vi "Execution_LaunchAnyProcess.vi"(7 "EVE reference in":refnum<data-value>, 8 "error in (no error)":errorcluster, 11 "Process in":refnum<class "Process.lvclass">) -> (0 "error out":errorcluster, 2 "vi reference":refnum<vi>, 3 "Process out":refnum<class "Process.lvclass">)   [LabVIEW 2013, in "Process.lvclass"]
uses:
  Process.lvclass
  001 - MAIN/Class/EVE/EVE.lvclass
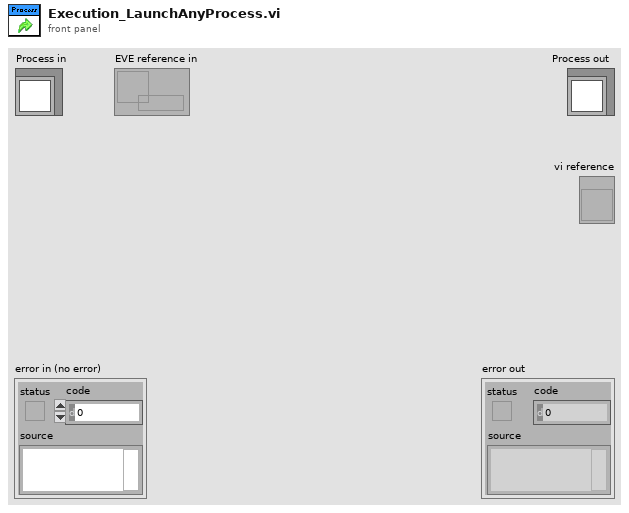
[diagram p1: front panel]
types:
  T1 = typedef "paramsExternalProcesses.ctl" = cluster{"Path":path, "Timeout":dbl, "viInitString":string, "State":enum32{"Invalid", "Standard", "Closed", "Hidden", "Minimized", "Maximized"}}
  T2 = enum32{"Invalid", "Standard", "Closed", "Hidden", "Minimized", "Maximized"}
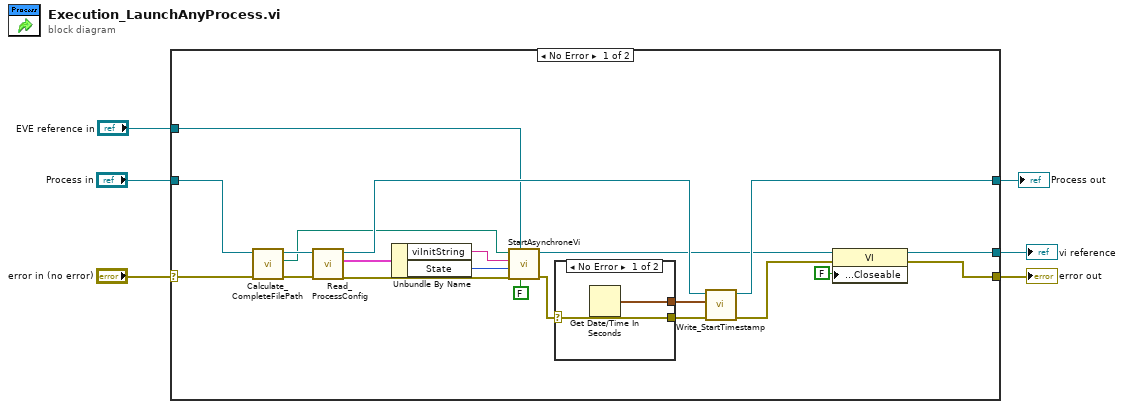
[diagram p0: block diagram]
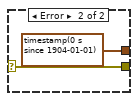
[diagram p2: hidden frame]
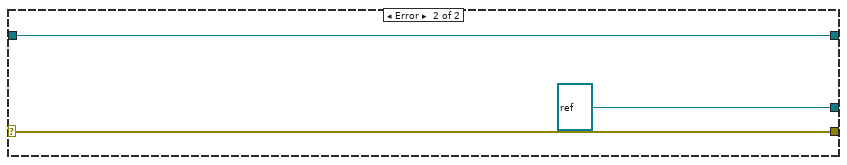
[diagram p3: hidden frame]
diagram:
  n1 = case shown="No Error" "error in (no error)" {
    selector: "error in (no error)" -> [w17 w34]
    tunnel: [w9 w34] -> w5
    tunnel: [w23 w33] -> w3
    tunnel: "Process in" -> [w14 w33]
    tunnel: [w11 refnum<vi> refnum ("vi reference")] -> w2
    tunnel: "EVE reference in" -> [w7 _]
    frame No Error {
      n2 = call-dynamic "Calculate_CompleteFilePath.vi"("error in"=w17, "Process in"=w14) -> ("error out"=w16:errorcluster, "Process Absolute Path"=w15:path, "Process out"=w18:refnum<class "Process.lvclass">)  [unwired: 7 in]
      n3 = call-dynamic "Read_ProcessConfig.vi"("error in (no error)"=w16, "Process in"=w18) -> ("error out"=w19:errorcluster, "ProcessConfig"=w27:T1, "Process out"=w24:refnum<class "Process.lvclass">)  [unwired: 7 in]
      n4 = Unbundle By Name(w27) -> ("viInitString"=w25:string, "State"=w26:T2)
      n5 = call "StartAsynchroneVi.vi"("Open Front Panel ?"=FALSE, "EVE reference in"=w7, "error in"=w19, "State"=w26, "viInitString"=w25, "viPathToStart"=w15) -> ("error out"=w21:errorcluster, "vi reference"=w12:refnum<vi>)  [unwired: 4 in]
      n6 = case shown="No Error" w21 {
        selector: w21 -> [w28 w31]
        tunnel: [w29 timestamp(0 s since 1904-01-01) ("seconds since 1Jan1904")] -> w22
        tunnel: [w28 w31] -> w20
        frame No Error {
          n7 = Get Date/Time In Seconds() -> (seconds since 1Jan1904=w29:timestamp)
        }
        frame Error {
        }
      }
      n8 = call-dynamic "Write_StartTimestamp.vi"("error in (no error)"=w20, "Start Timestamp"=w22, "Process in"=w24) -> ("error out"=w10:errorcluster, "Process out"=w23:refnum<class "Process.lvclass">)  [unwired: 7 in]
      n9 = property class="VI"(reference=w12, error in=w10, "Front Panel.Closeable"=FALSE ("Front Panel Window:Closeable")) -> (reference out=w11:refnum<vi>, error out=w9:errorcluster)
    }
    frame Error {
    }
  }
  "error out" <- w5
  "Process out" <- w3
  "vi reference" <- w2
